vi "Parse Channels.vi"(8 "error in (no error)":errorcluster, 9 "Specified Channel Ref List":T1[](array[typedef]) format="%.0x", 10 "Section GUID":string, 11 "Device Reference in":T1 format="%.0x") -> (0 "error out":errorcluster, 1 "Section BaseRate":i32, 2 "Channel Data []":T2[](array[typedef]) {"Labels Settings"."Word"."Param Setting"."Num Bits" min=1 max=32; "Labels Settings"."Word"."Param Setting"."Start Bit" min=8 max=31; "Labels Settings"."Label" format="%.0o"}, 3 "Device Reference out":T1 format="%.0x")   [LabVIEW 2017, in "Ballard Arinc-429 System Explorer.lvlib"]
uses:
  System Explorer/Ballard Arinc-429 System Explorer.lvlib
  RT Controls/RT HW Channel.ctl
  RT Controls/RT Label Settings.ctl
  Shared/Controls and Global/Label.ctl
  Shared/Controls and Global/transferPeriod.ctl
  RT Controls/RT Word Settings.ctl
  RT Controls/RT Param Setting.ctl
  Shared/Controls and Global/Start Bit.ctl
  Shared/Controls and Global/Number of Bits.ctl
  Shared/Controls and Global/TransferType.ctl
  <vilib>/NI Veristand/Custom Device API/Custom Device Item Ref.ctl
  <vilib>/NI Veristand/Custom Device API/Get Item Property (U16).vi
  Shared/Controls and Global/Global.vi
  <vilib>/NI Veristand/Custom Device Tools/Custom Device Utility Library/NI VeriStand - Search for Item by GUID.vi
  <vilib>/NI Veristand/Custom Device Tools/Custom Device Utility Library/Custom Device Utility Library.lvlib
  <vilib>/NI Veristand/Custom Device API/Custom Device API.lvlib
  Shared/Ballard Arinc-429 Shared.lvlib
  Ballard Arinc-429 Engine.lvlib
  <vilib>/NI Veristand/Custom Device API/Get Item Property (Double).vi
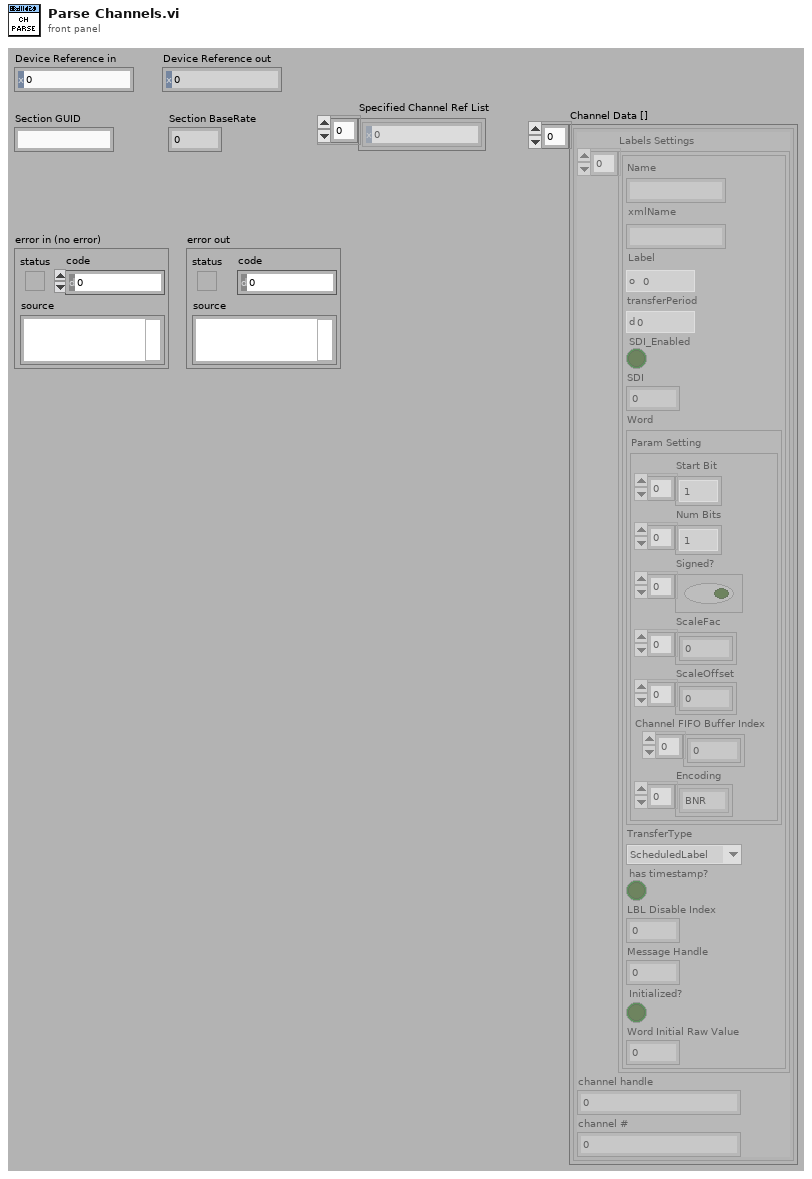
[diagram p1: front panel]
types:
  T1 = typedef "Custom Device API.lvlib/Custom Device Item Ref.ctl" = u64
  T2 = typedef "Ballard Arinc-429 Engine.lvlib/RT HW Channel.ctl" = cluster{"Labels Settings":T3[], "channel handle":u32, "channel #":u16}
  T3 = typedef "Ballard Arinc-429 Engine.lvlib/RT Label Settings.ctl" = cluster{"Name":string, "xmlName":string, "Label":T4, "transferPeriod":T5, "SDI_Enabled":bool, "SDI":u8, "Word":T6, "TransferType":T10, "has timestamp?":bool, "LBL Disable Index":i32, "Message Handle":u64, "Initialized?":bool, "Word Initial Raw Value":u32}
  T4 = typedef "Ballard Arinc-429 Shared.lvlib/Label.ctl" = u8
  T5 = typedef "Ballard Arinc-429 Shared.lvlib/transferPeriod.ctl" = u32
  T6 = typedef "Ballard Arinc-429 Engine.lvlib/RT Word Settings.ctl" = cluster{"Param Setting":T7}
  T7 = typedef "Ballard Arinc-429 Engine.lvlib/RT Param Setting.ctl" = cluster{"Start Bit":T8[], "Num Bits":T9[], "Signed?":bool[], "ScaleFac":dbl[], "ScaleOffset":dbl[], "Channel FIFO Buffer Index":i32[], "Encoding":enum16{"BNR", "BCD", "Discrete"}[]}
  T8 = typedef "Ballard Arinc-429 Shared.lvlib/Start Bit.ctl" = i32
  T9 = typedef "Ballard Arinc-429 Shared.lvlib/Number of Bits.ctl" = i32
  T10 = typedef "Ballard Arinc-429 Shared.lvlib/TransferType.ctl" = enum16{"ScheduledLabel", "Acyclic", "Block", "Strobe"}
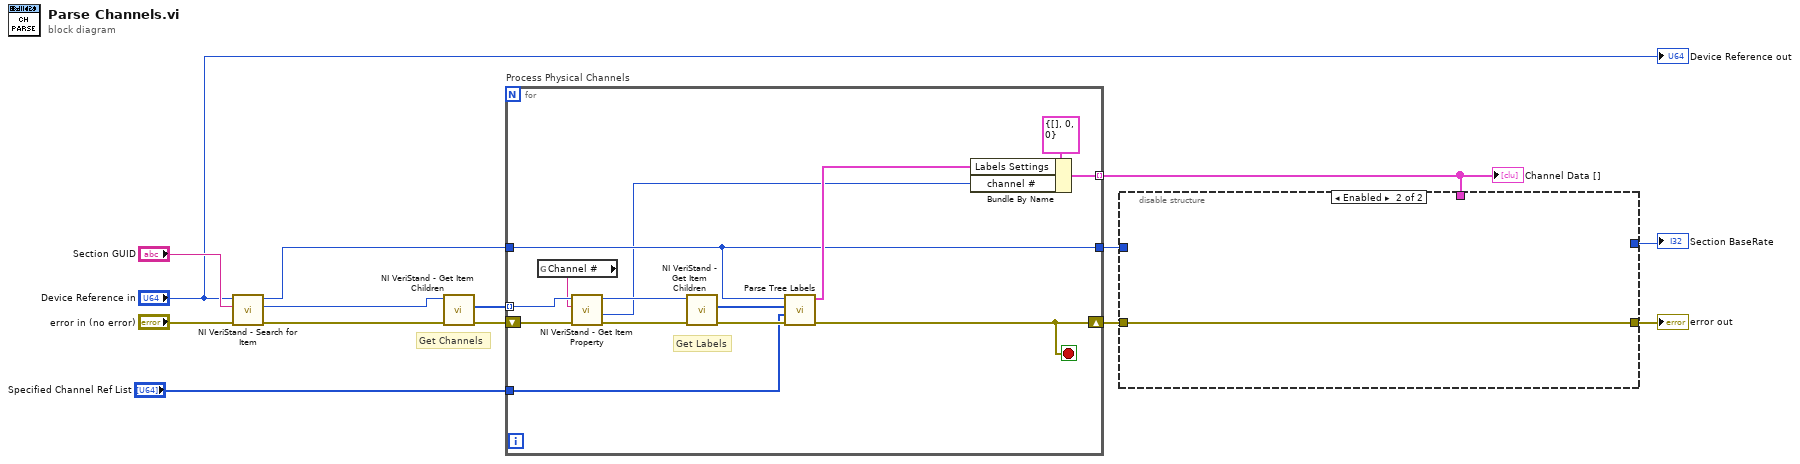
[diagram p0: block diagram]
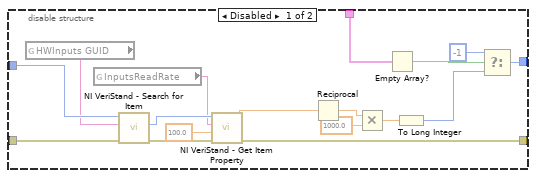
[diagram p2: hidden frame]
diagram:
  # "Get Channels"
  n1 = call-poly <vilib>:"NI VeriStand - Search for Item.vi"("error in"="error in (no error)", "Item GUID"="Section GUID", "Section Ref in"="Device Reference in") -> ("error out"=w9:errorcluster, "Item Ref"=w10:T1, "Section Ref out"=w14:T1)  [unwired: 5 in, 1 out]
  n2 = call <vilib>:"NI VeriStand - Get Item Children.vi"("error in (no error)"=w9, "Item Ref in"=w10) -> ("error out"=w13:errorcluster, "Child Refs"=w12:T1[])  [unwired: 6 in, 2 out]
  n3 = for "Process Physical Channels" {
    tunnel: w12 -> [w22] mode=indexing
    tunnel: w14 -> [w20]
    tunnel: [w26] -> w6 mode=indexing
    shift-right: [w16] -> w4
    shift-left: w13 -> [w24]
    tunnel: [w20] -> w3
    tunnel: "Specified Channel Ref List" -> [w15]
    stop <- w16 stop-if-true
    # "Get Labels"
    n4 = global read "Global.vi" "Channel #"() -> (w18:string)
    n5 = call-poly <vilib>:"NI VeriStand - Get Item Property.vi"("error in (no error)"=w24, "Property Name"=w18, "Item Ref in"=w22) -> ("error out"=w23:errorcluster, "Value"=w17:u16, "Item Ref out"=w21:T1)  [unwired: 5 in, 1 out]
    n6 = call <vilib>:"NI VeriStand - Get Item Children.vi"("error in (no error)"=w23, "Item Ref in"=w21) -> ("error out"=w25:errorcluster, "Child Refs"=w19:T1[])  [unwired: 6 in, 2 out]
    n7 = call "Parse Tree Labels.vi"("error out"=w25, "Specified Channel Ref List"=w15, "Label Refs"=w19, "Custom Device Ref"=w20) -> ("error out"=w16:errorcluster, "Label data"=w27:T3[])  [unwired: 6 in]
    n8 = Bundle By Name(cluster=T2 {"Labels Settings"=[], "channel handle"=0, "channel #"=0} ("HW Channel"), "Labels Settings"=w27, "channel #"=w17) -> (w26:T2)
  }
  "Channel Data []" <- w6
  n9 = disable-structure shown="Enabled" {
    disable-tunnel: [w45 _] -> w7
    disable-tunnel: w6 -> [w44 _]
    disable-tunnel: [w43 w46] -> w5
    disable-tunnel: w4 -> [w42 w46]
    disable-tunnel: w3 -> [w41 _]
    frame Disabled {
      n10 = global read "Global.vi" "HWInputs GUID"() -> (w40:string)
      n11 = global read "Global.vi" "InputsReadRate"() -> (w37:string)
      n12 = call-poly <vilib>:"NI VeriStand - Search for Item.vi"("error in"=w42, "Item GUID"=w40, "Section Ref in"=w41) -> ("error out"=w39:errorcluster, "Item Ref"=w38:T1)  [unwired: 5 in, 2 out]
      n13 = call-poly <vilib>:"NI VeriStand - Get Item Property.vi"("error in (no error)"=w39, "Default Value"=100.0, "Property Name"=w37, "Item Ref in"=w38) -> ("error out"=w43:errorcluster, "Value"=w36:dbl)  [unwired: 4 in, 2 out]
      n14 = Reciprocal(x=w36) -> (1/x=w34:dbl)
      n15 = Multiply(x=w34, y=1000.0) -> (x*y=w32:dbl)
      n16 = Empty Array?(array=w44) -> (empty?=w30:bool)
      n17 = To Long Integer(number=w32) -> (32bit integer=w29:i32)
      n18 = Select(t=-1, s=w30, f=w29) -> (s? t:f=w45:i32)
    }
    frame Enabled {
    }
  }
  "error out" <- w5
  "Section BaseRate" <- w7
  "Device Reference out" <- "Device Reference in"
